vi "Mappa DO PLC_2.vi"(11 "USCITE PLC 2":T1={"AO (real) 2"={"SCORTA 1"=0.0, "SCORTA 2"=0.0, "SCORTA 3"=0.0, "SCORTA 4"=0.0, "SCORTA 5"=0.0, "SCORTA 6"=0.0, "SCORTA 7"=0.0, "SCORTA 8"=0.0}, "statoAO_PLC out"={"Condensatori"=nan, "Scorta 1"=nan, "Scorta 2"=0.0}, "DO (bit)"={"Relè misura resistomat"=FALSE, "Misura res ramo 1"=FALSE, "Misura res ramo 2"=FALSE, "Misura res ramo 3"=FALSE, "Scelta banco 2"=FALSE, "Scala Torsiometro"=FALSE, "Ctrl torsiometro"=FALSE, "Select current mode"=FALSE, "Select Torque mode"=FALSE, "Select speed mode"=FALSE, "Watchdog"=FALSE, "Scorta"=FALSE, "Scorta 2"=FALSE, "Scorta 3"=FALSE, "Scorta 4"=FALSE, "Scorta 5"=FALSE, "Bench selection"=FALSE, "External alarm"=FALSE, "Enable external program"=FALSE, "Reset allarmi"=FALSE, "Start"=FALSE, "Stop"=FALSE, "Block"=FALSE, "Scorta 6"=FALSE}}) -> (1 "DO (DATABLOCK)":bool[](array[boolean]), 3 "DO (MERKER)":bool[](array[boolean]))   [LabVIEW 2019]
uses:
  Uscite PLC 2.ctl
  controls/statoAO_plc_2.ctl
  StatoDO_PLC_2.ctl
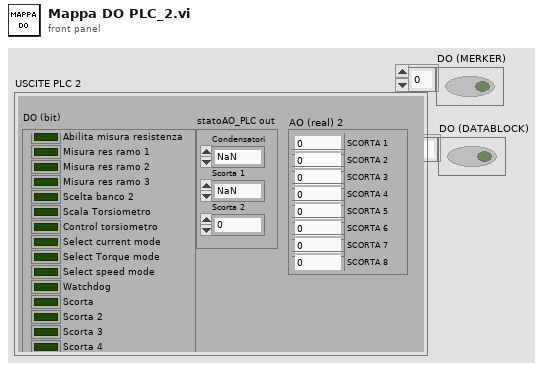
[diagram p1: front panel]
types:
  T1 = typedef "Uscite PLC 2.ctl" = cluster{"AO (real) 2":cluster{"SCORTA 1":dbl, "SCORTA 2":dbl, "SCORTA 3":dbl, "SCORTA 4":dbl, "SCORTA 5":dbl, "SCORTA 6":dbl, "SCORTA 7":dbl, "SCORTA 8":dbl}, "statoAO_PLC out":T2, "DO (bit)":T3}
  T2 = typedef "statoAO_plc_2.ctl" = cluster{"Condensatori":dbl, "Scorta 1":dbl, "Scorta 2":dbl}
  T3 = typedef "StatoDO_PLC_2.ctl" = cluster{"Relè misura resistomat":bool, "Misura res ramo 1":bool, "Misura res ramo 2":bool, "Misura res ramo 3":bool, "Scelta banco 2":bool, "Scala Torsiometro":bool, "Ctrl torsiometro":bool, "Select current mode":bool, "Select Torque mode":bool, "Select speed mode":bool, "Watchdog":bool, "Scorta":bool, "Scorta 2":bool, "Scorta 3":bool, "Scorta 4":bool, "Scorta 5":bool, "Bench selection":bool, "External alarm":bool, "Enable external program":bool, "Reset allarmi":bool, "Start":bool, "Stop":bool, "Block":bool, "Scorta 6":bool}
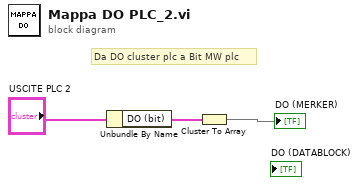
[diagram p0: block diagram]
diagram:
  # "Da DO cluster plc a Bit MW plc"
  n1 = Unbundle By Name("USCITE PLC 2") -> ("DO (bit)"=w2:T3)
  n2 = Cluster To Array(cluster=w2) -> (array=→"DO (MERKER)":bool[])
